vi "Qr.vi"() -> ()   [LabVIEW 2017]
uses:
  <vilib>/vision/Instrument.llb/QR Code Description Options.ctl
  <vilib>/vision/Instrument.llb/Data Matrix Polarity.ctl
  <vilib>/vision/Instrument.llb/QR Code Model Type.ctl
  <vilib>/Utility/config.llb/Read Key (String).vi
  <vilib>/Utility/config.llb/Write Key (String).vi
  <vilib>/regexp/Match Regular Expression.xnode
  <vilib>/vision/driver/NI_Vision_Acquisition_Software.lvlib
  <vilib>/Utility/config.llb/NI_LVConfig.lvlib
  <vilib>/vision/NI_Vision_Development_Module.lvlib
panel:
  in  "Analyze":bool
  in  "Clipboard":bool
  out "Image":T1(plugin-control)
  in  "stop":bool
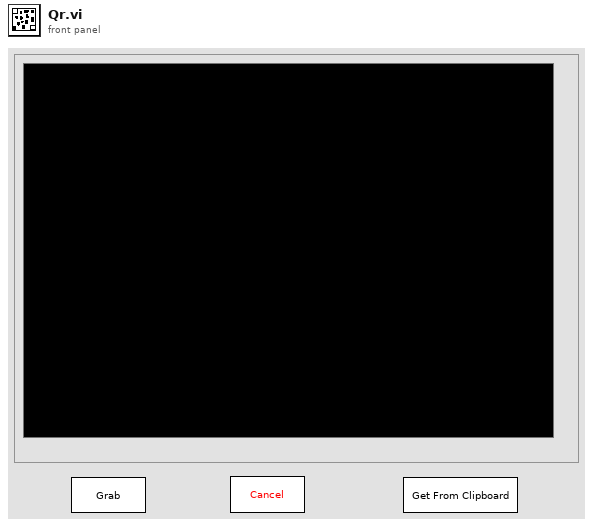
[diagram p1: front panel]
types:
  T1 = typedef "IMAQ Image.ctl" = refnum<image>
  T2 = typedef "Image Type" = u32
  T3 = typedef "NI_LVConfig.lvlib/Config Data RefNum.ctl" = refnum<k1>
  T4 = typedef "IMAQdx.ctl" = refnum<k21>
  T5 = typedef "QR Code Description Options.ctl" = cluster{"Matrix Size (cells)":i32, "Barcode Polarity":T6, "Mirror Mode":i32, "QR Model":T7}
  T6 = typedef "Data Matrix Polarity.ctl" = i32
  T7 = typedef "QR Code Model Type.ctl" = i32
  T8 = cluster{"Rotation Mode":enum32{"Unlimited", "0 Degrees", "90 Degrees", "180 Degrees", "270 Degrees"}, "Skip Location?":bool, "Edge Threshold":u32, "Demodulation Mode":i32, "Cell Sample Size":i32, "Cell Filter Mode":i32, "Skew Degrees Allowed":u32}
  T9 = cluster{"Global Rectangle":i32[], "Contours":cluster{"ID":enum32{"External", "Internal"}, "Type":u32, "Coordinates":i32[]}[]}
  T10 = typedef "QR Code Report.ctl" = cluster{"Found?":bool, "Data":string, "Bounding Box":cluster{"x":sgl, "y":sgl}[], "Errors Corrected":u32, "Dimensions (Rows/Cols)":u32, "Version":u32, "QR Model":T7, "Stream Mode":T11, "Barcode Polarity":T6, "Mirrored?":bool, "Append Stream Position":u32, "Size of Append Stream":u32, "First EAN-128 ID":i32, "First Alternate Language ID":i32, "Append Stream ID":u32, "Minimum Edge Strength":u32, "Demodulation Mode":T12, "Cell Sample Size":T13, "Cell Filter Mode":T14}
  T11 = typedef "QR Code Stream Mode Type.ctl" = i32
  T12 = typedef "Demodulation Mode.ctl" = i32
  T13 = typedef "Cell Sample Size.ctl" = i32
  T14 = typedef "Cell Filter Mode.ctl" = i32
  T15 = cluster{"trimmed string":string, "trimmed string":string}
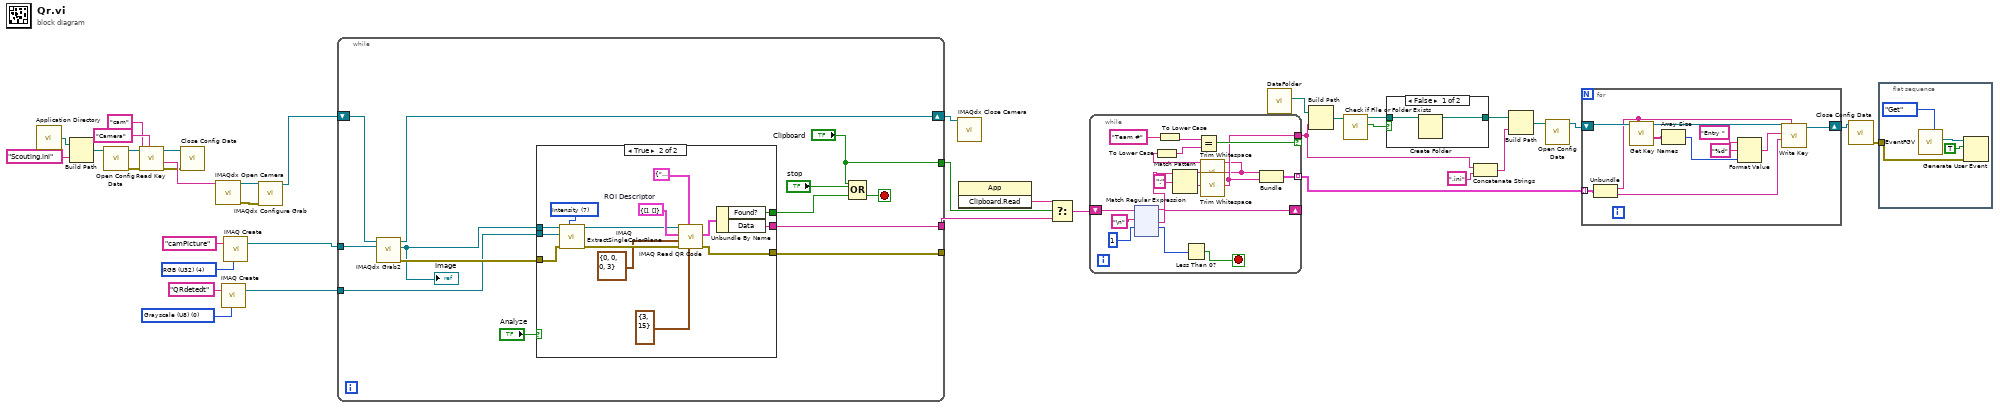
[diagram p0: block diagram]
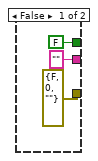
[diagram p2: hidden frame]
diagram:
  w33 = T2 0 items=["Grayscale (U8)", "Grayscale (I16)", "Grayscale (SGL)", "Complex (CSG)", "RGB (U32)", "HSL (U32)", "RGB (U64)", "Grayscale (U16)"] ("Image Type")
  w34 = T2 4 items=["Grayscale (U8)", "Grayscale (I16)", "Grayscale (SGL)", "Complex (CSG)", "RGB (U32)", "HSL (U32)", "RGB (U64)", "Grayscale (U16)"] ("Image Type")
  n1 = call <vilib>:"Application Directory.vi"() -> ("Application Directory"=w17:path)
  n2 = Build Path(base path=w17, name or relative path="Scouting.ini") -> (appended path=w15:path)
  n3 = call <vilib>:"Open Config Data.vi"("configuration file path"=w15) -> ("error out"=w14:errorcluster, "refnum"=w13:T3)  [unwired: 8 in, 1 out]
  n4 = call-poly <vilib>:"Read Key.vi"("section"="Camera", "error in (no error)"=w14, "key"="cam", "refnum"=w13) -> ("error out"=w10:errorcluster, "value"=w32:string, "refnum out"=w9:T3)  [unwired: 4 in, 1 out]
  n5 = call <vilib>:"Close Config Data.vi"("error in (no error)"=w10, "refnum"=w9) -> ()  [unwired: 8 in, 2 out]
  n6 = call <vilib>:"IMAQdx Open Camera.vi"("Session In"=w32) -> ("error out"=w31:errorcluster, "Session Out"=w36:T4)  [unwired: 9 in]
  n7 = call "IMAQ Create"("Image Name"="QRdetedt", "Image Type"=w33) -> ("New Image"=w6:T1)  [unwired: 3 in, 1 out]
  n8 = call "IMAQ Create"("Image Name"="camPicture", "Image Type"=w34) -> ("New Image"=w7:T1)  [unwired: 3 in, 1 out]
  n9 = call <vilib>:"IMAQdx Configure Grab.vi"("error in"=w31, "Session In"=w36) -> ("Session Out"=w8:T4)  [unwired: 8 in, 1 out]
  n10 = while {
    tunnel: [w50] -> _
    tunnel: [w49] -> w4
    shift-right: [w48] -> w5
    shift-left: w8 -> [w46]
    tunnel: w6 -> [w42]
    tunnel: w7 -> [w47]
    tunnel: ["Clipboard"] -> w2
    stop <- w43 stop-if-true
    n11 = call <vilib>:"IMAQdx Grab2.vi"("Image In"=w47, "Session In"=w46) -> ("error out"=w45:errorcluster, "Image Out"=w41:T1, "Session Out"=w48:T4)  [unwired: 6 in, 1 out]
    "Image" <- w41
    n12 = case shown="True" "Analyze" {
      tunnel: [errorcluster {"status"=FALSE, "code"=0, "source"=""} ("error out") w62] -> w50
      tunnel: ["" ("Data") w60] -> w49
      tunnel: w45 -> [_ w59]
      tunnel: [FALSE ("Found?") w58] -> w44
      tunnel: w42 -> [_ w57]
      tunnel: w41 -> [_ w54]
      frame False {
      }
      frame True {
        w63 = T9 {"Global Rectangle"=[], "Contours"=[]}  # ROI Descriptor
        w67 = 7 items=["Red", "Green", "Blue", "Hue", "Saturation", "Luminance", "Value", "Intensity"] ("Color Plane")
        n13 = call "IMAQ ExtractSingleColorPlane"("Color Plane"=w67, "error in (no error)"=w59, "Image Dst"=w57, "Image Src"=w54) -> ("error out"=w66:errorcluster, "Image Dst Out"=w56:T1)  [unwired: 6 out]
        n14 = call "IMAQ Read QR Code"("QR Code Cell Size (pixels)"=cluster{"Minimum Size":u32, "Maximum Size":u32} {"Minimum Size"=3, "Maximum Size"=15}, "QR Search Options"=T8 {"Rotation Mode"=enum."Unlimited", "Skip Location?"=FALSE, "Edge Threshold"=30, "Demodulation Mode"=-2, "Cell Sample Size"=-2, "Cell Filter Mode"=-2, "Skew Degrees Allowed"=15}, "error in (no error)"=w66, "QR Description Options"=T5 {"Matrix Size (cells)"=0, "Barcode Polarity"=0, "Mirror Mode"=0, "QR Model"=3}, "ROI Descriptor"=w63, "Image"=w56) -> ("error out"=w62:errorcluster, "QR Code Report"=w61:T10)  [unwired: 1 in, 3 out]
        n15 = Unbundle By Name(w61) -> ("Found?"=w58:bool, "Data"=w60:string)
      }
    }
    n16 = Compound Arithmetic op=OR("Clipboard", "stop", w44) -> (w43:bool)
  }
  n17 = call <vilib>:"IMAQdx Close Camera.vi"("Session In"=w5) -> ()  [unwired: 10 in, 1 out]
  n18 = invoke class="App" method="Clipboard.Read"() -> ("Read Clipbrd"=w1:string)  [unwired: 3 in, 2 out]
  n19 = Select(t=w1, s=w2, f=w4) -> (s? t:f=w3:string)
  n20 = while {
    shift-right: [w84] -> _
    shift-left: w3 -> [w71]
    tunnel: [w77] -> w20 mode=indexing
    tunnel: [w69] -> w27 if=w72
    stop <- w80 stop-if-true
    n21 = xnode "Match Regular Expression"("input string"=w71, "regular expression"="\n" ("search string/char (-)"), "offset (0)"=1) -> ("before match"=w70:string, "after match"=w84:string, "offset past match"=w81:i32)  [unwired: 3 in, 2 out]
    n22 = To Lower Case(string="Team #") -> (all lower case string=w75:string)
    n23 = Match Pattern(string=w70, regular expression=":" ("search string/char (-)")) -> (before substring=w78:string, after substring=w73:string)  [unwired: 1 in, 2 out]
    n24 = Less Than 0?(x=w81) -> (x < 0?=w80:bool)
    n25 = call <vilib>:"Trim Whitespace.vi"("string"=w78) -> ("trimmed string"=w68:string)  [unwired: 1 in]
    n26 = To Lower Case(string=w68) -> (all lower case string=w74:string)
    n27 = Equal?(x=w75, y=w74) -> (x = y?=w72:bool)
    n28 = call <vilib>:"Trim Whitespace.vi"("string"=w73) -> ("trimmed string"=w69:string)  [unwired: 1 in]
    n29 = Bundle("trimmed string"=w68, "trimmed string"=w69) -> (w77:T15)  [unwired: 1 in]
  }
  n30 = call "DataFolder.vi"() -> ("appended path"=w29:path)  [unwired: 11 in]
  n31 = Build Path(base path=w29, name or relative path=w27) -> (appended path=w28:path)
  n32 = call <vilib>:"Check if File or Folder Exists.vi"("path"=w28) -> ("file or folder exists?"=w23:bool, "dup path"=w30:path)  [unwired: 8 in, 1 out]
  n33 = case shown="False" w23 {
    tunnel: w30 -> [w200 w201]
    tunnel: [w199 w201] -> w25
    frame False {
      n34 = Create Folder(path (use dialog)=w200) -> (created path=w199:path)  [unwired: 2 in, 2 out]
    }
    frame True {
    }
  }
  n35 = Concatenate Strings(w27, ".ini" ("format string")) -> (w24:string)
  n36 = Build Path(base path=w25, name or relative path=w24) -> (appended path=w22:path)
  n37 = call <vilib>:"Open Config Data.vi"("configuration file path"=w22) -> ("refnum"=w21:T3)  [unwired: 8 in, 2 out]
  n38 = for {
    tunnel: w20 -> [w211] mode=indexing
    shift-right: [w202] -> w19
    shift-left: w21 -> [w212]
    n39 = Unbundle(w211) -> ("trimmed string"=w209:string, "trimmed string"=w208:string)
    n40 = call <vilib>:"Get Key Names.vi"("section"=w209, "refnum"=w212) -> ("key names"=w210:string[], "refnum out"=w207:T3)  [unwired: 6 in, 2 out]
    n41 = Array Size(array=w210) -> (size(s)=w205:i32)
    n42 = Format Value(string ("")="Entry ", format string="%d", value (0)=w205) -> (output string=w203:string)
    n43 = call-poly <vilib>:"Write Key.vi"("section"=w209, "value"=w208, "key"=w203, "refnum"=w207) -> ("refnum out"=w202:T3)  [unwired: 5 in, 2 out]
  }
  n44 = call <vilib>:"Close Config Data.vi"("refnum"=w19) -> ("error out"=w18:errorcluster)  [unwired: 9 in, 1 out]
  n45 = flat-sequence {
    tunnel: w18 -> [w213]
    frame #0 {
      n46 = call "EventFGV.vi"("Action"=enum16{"Set", "Get"}."Get") -> ("user event out"=w215:refnum<user-event>)  [unwired: 10 in]
      n47 = Generate User Event(user event=w215, event data cluster=TRUE ("event data"), error in=w213) -> ()  [unwired: 1 in, 2 out]
    }
  }
